vi "Periodic Tasks.vi"(8 "error in":errorcluster) -> ()   [LabVIEW 2017]
doc: "This VI runs in parallel to other robot code. It can contain as many user-defined periodic loops as you need. These can carry out PID or other sorts of timed response."
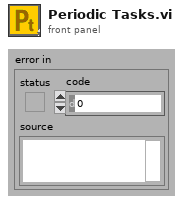
[diagram p1: front panel]
types:
  T1 = typedef "WPI_JoystickDevRef.ctl" = cluster{"Device":T2}
  T2 = typedef "WPI_JoystickDeviceEnum.ctl" = enum16{"USB 0", "USB 1", "USB 2", "USB 3", "USB 4", "USB 5"}
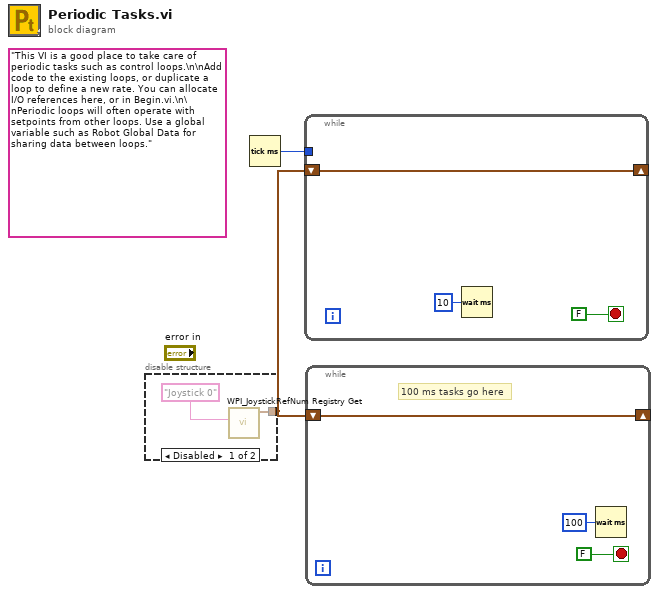
[diagram p0: block diagram]
diagram:
  (unwired) "This VI is a good place to take care of periodic tasks such as control loops.\n\nAdd code to the existing loops, or duplicate a loop to define a new rate. You can allocate I/O references here, or in Begin.vi.\n\nPeriodic loops will often operate with setpoints from other loops. Use a global variable such as Robot Global Data for sharing data between loops."
  n1 = disable-structure shown="Disabled" {
    disable-tunnel: [w3 _] -> w2
    frame Disabled {
      n2 = call <vilib>:"WPI_JoystickRefNum Registry Get.vi"("refnum name"="Joystick 0") -> ("JoystickDevRef"=w3:T1)  [unwired: 1 in, 9 out]
    }
    frame Enabled {
    }
  }
  n3 = Tick Count (ms)() -> (millisecond timer value=w1:u32)
  n4 = while {
    shift-right: [w6] -> _
    shift-left: w2 -> [w6]
    tunnel: w1 -> [_]
    stop <- FALSE stop-if-true
    n5 = Wait (ms)(milliseconds to wait=u32 10) -> ()  [unwired: 1 out]
  }
  n6 = while {
    shift-right: [w8] -> _
    shift-left: w2 -> [w8]
    stop <- FALSE stop-if-true
    # "100 ms tasks go here"
    n7 = Wait (ms)(milliseconds to wait=u32 100) -> ()  [unwired: 1 out]
  }
